vi "LoopComp.vi"(2 "RandTime":u64 caption="Rand Time (ms)", 3 "LoopPeriod":u64=1 caption="Loop Period (ms)", 4 "SetTime":u64=1000 caption="Set Time (ms)", 6 "LoopCount":u64, 7 "Mode":enum16{"Reset", "Run"}(ring)) -> (0 "ActualTime":u64=1000 caption="Actual Time (ms)", 1 "Outcome":enum16{"TimeIn", "TimeOut"}(ring))   [LabVIEW 2011]
panel:
  out "RandCount":dbl=1.0
  out "SetCount":dbl=1.0
  in  "BaseCount":u64
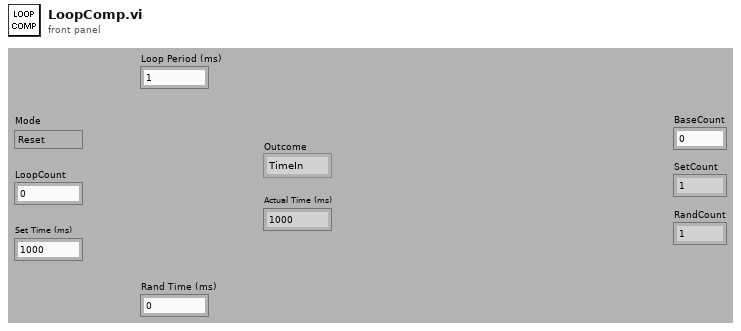
[diagram p1: front panel]
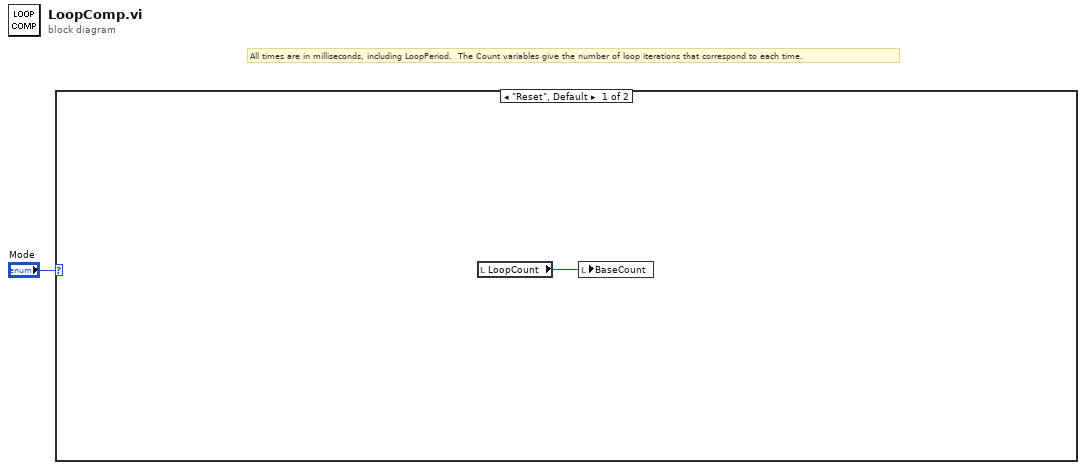
[diagram p0: block diagram]
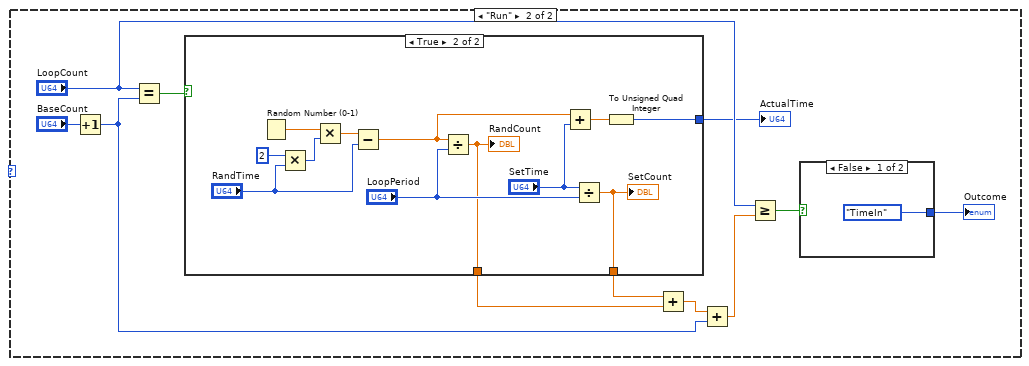
[diagram p2: hidden frame]
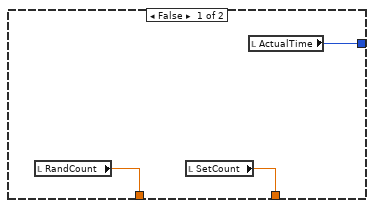
[diagram p3: hidden frame]
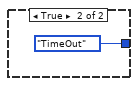
[diagram p4: hidden frame]
diagram:
  # "All times are in milliseconds, including LoopPeriod.  The Count variables give the number of loop iterations that correspond to each time."
  n1 = case shown="\"Reset\", Default" "Mode" {
    frame "Reset", Default {
      n2 = local read "LoopCount"() -> (w2:u64)
      n3 = local write "BaseCount"(w2) -> ()
    }
    frame "Run" {
      n4 = Increment(x="BaseCount") -> (x+1=w4:u64)
      n5 = Equal?(x="LoopCount", y=w4) -> (x = y?=w10:bool)
      n6 = case shown="True" w10 {
        tunnel: [w15 w20] -> w8
        tunnel: [w16 w19] -> w7
        tunnel: [w14 w17] -> w3
        frame False {
          n7 = local read "RandCount"() -> (w16:dbl)
          n8 = local read "SetCount"() -> (w15:dbl)
          n9 = local read "ActualTime"() -> (w14:u64)
        }
        frame True {
          n10 = Random Number (0-1)() -> (number: 0 to 1=w28:dbl)
          n11 = Multiply(x=u64 2 ("y"), y="RandTime") -> (x*y=w27:u64)
          n12 = Multiply(x=w28, y=w27) -> (x*y=w26:dbl)
          n13 = Subtract(x=w26, y="RandTime") -> (x-y=w21:dbl)
          n14 = Divide(x=w21, y="LoopPeriod") -> (x/y=w19:dbl)
          "RandCount" <- w19
          n15 = Add(x=w21, y="SetTime") -> (x+y=w18:dbl)
          n16 = Divide(x="SetTime", y="LoopPeriod") -> (x/y=w20:dbl)
          "SetCount" <- w20
          n17 = To Unsigned Quad Integer(1:w18) -> (0:w17:u64)
        }
      }
      "ActualTime" <- w3
      n18 = Add(x=w8, y=w7) -> (x+y=w12:dbl)
      n19 = Add(x=w12, y=w4) -> (x+y=w11:dbl)
      n20 = Greater Or Equal?(x="LoopCount", y=w11) -> (x >= y?=w13:bool)
      n21 = case shown="False" w13 {
        tunnel: [enum16{"TimeIn", "TimeOut"}."TimeIn" ("Outcome") enum16{"TimeIn", "TimeOut"}."TimeOut" ("Outcome")] -> w6
        frame False {
        }
        frame True {
        }
      }
      "Outcome" <- w6
    }
  }
